vi "JIL-XML.vi"() -> ()   [LabVIEW 2010]
panel:
  in  "UseAuthentication":bool
  in  "MaxClients":i32=6
  out "clients":i32
  out "RegText":string
  in  "OpenFP":bool=TRUE
  out "error out 2":errorcluster={"status"=TRUE, "code"=56, "source"="TCP Wait On Listener in JIL-XML.vi"}
  in  "OpenParser":bool=TRUE
  out "error out":errorcluster
  out "Error":errorcluster={"status"=TRUE, "code"=56, "source"="TCP Wait On Listener in JIL-XML.vi"}
  in  "stop":bool=TRUE
  out "remote address":string
  in  "port":u16=2055
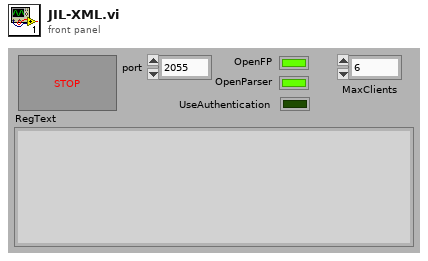
[diagram p1: front panel]
types:
  T1 = enum16{"Update", "registry", "Init", "clean", "Close"}
  T2 = enum32{"Invalid", "Standard", "Closed", "Hidden", "Minimized", "Maximized"}
  T3 = cluster{"remote address":string, "remote port":u16}
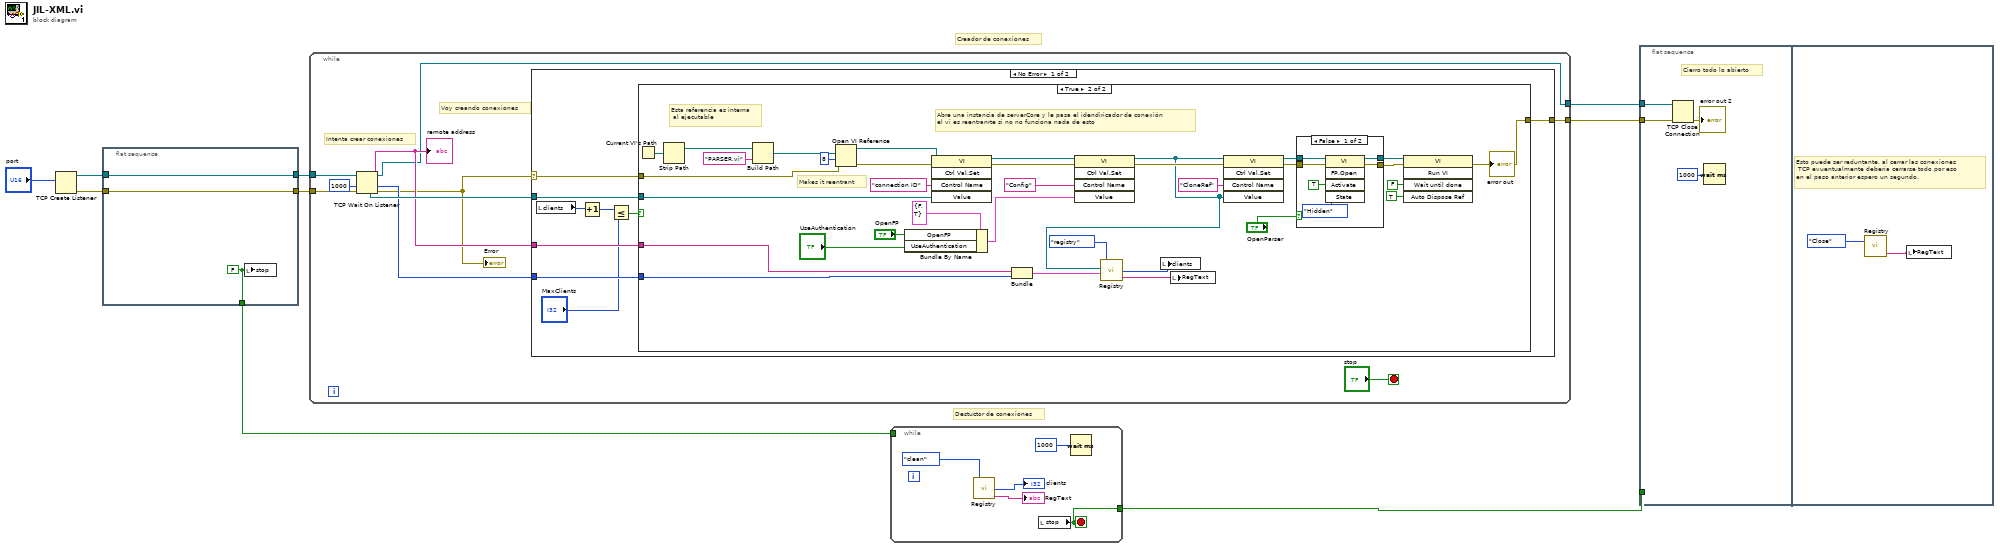
[diagram p0: block diagram]
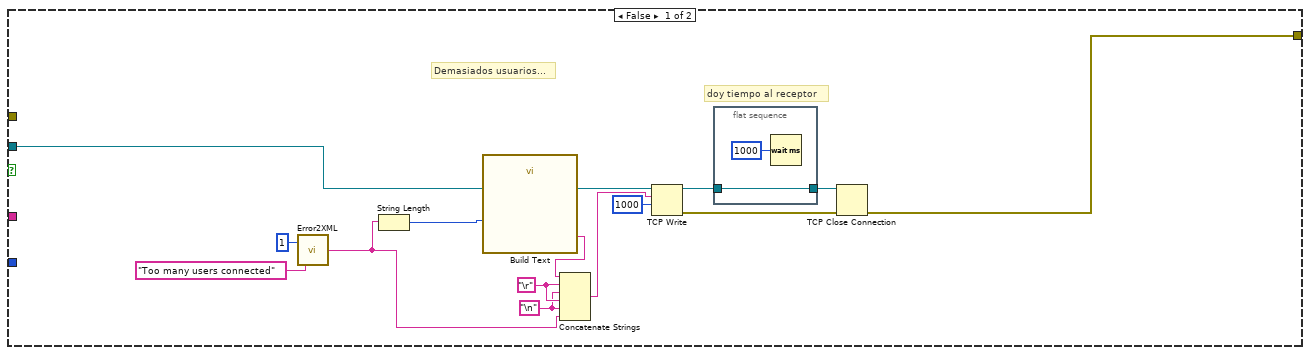
[diagram p2: hidden frame]
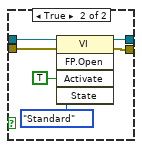
[diagram p3: hidden frame]
diagram:
  # "Destuctor de conexiones"
  # "Creador de conexiones"
  n1 = TCP Create Listener(10:"port") -> (0:w6:errorcluster, 3:w7:refnum<k5>)  [unwired: 4 in, 1 out]
  n2 = flat-sequence {
    tunnel: [w12] -> w8
    tunnel: w7 -> [w12]
    tunnel: w6 -> [w11]
    tunnel: [w11] -> w5
    tunnel: [w10] -> w3
    frame #0 {
      w10 = FALSE ("stop")
      n3 = local write "stop"(w10) -> ()
    }
  }
  n4 = while {
    tunnel: w8 -> [w15]
    tunnel: w5 -> [w22]
    tunnel: [w14] -> w1
    tunnel: [w18] -> w2
    stop <- "stop" stop-if-true
    # "Intenta crear conexiones"
    # "Voy creando conexiones"
    n5 = TCP Wait On Listener(8:w22, 9:1000 ("timeout ms (wait forever: -1)"), 11:w15) -> (0:w13:errorcluster, 1:w16:u16, 2:w17:string, 3:w14:refnum<k5>, 4:w21:refnum<k5>)  [unwired: 1 in]
    "remote address" <- w17
    "Error" <- w13
    n6 = case shown="No Error" w13 {
      selector: w13 -> [w27 w94]
      tunnel: w21 -> [w31 _]
      tunnel: [w30 w94] -> w18
      tunnel: w17 -> [w29 _]
      tunnel: w16 -> [w28 _]
      frame No Error {
        n7 = local read "clients"() -> (w24:i32)
        n8 = Increment(x=w24) -> (x+1=w25:i32)
        n9 = Less Or Equal?(x=w25, y="MaxClients") -> (x <= y?=w26:bool)
        n10 = case shown="True" w26 {
          tunnel: w31 -> [w42 w80]
          tunnel: [w40 w73] -> w30
          tunnel: w29 -> [_ w52]
          tunnel: w28 -> [_ w51]
          tunnel: w27 -> [_ w49]
          frame False {
            w34 = "\n"
            w35 = "\r"
            # "doy tiempo al receptor"
            # "Demasiados usuarios..."
            n11 = call "Error2XML.vi"("FailDescriptor"="Too many users connected", "FailID"=1) -> ("ErrorXML"=w32:string)
            n12 = String Length(string=w32) -> (length=w37:i32)
            n13 = call "Build Text"("longitud"=w37) -> ("Result"=w36:string)  [unwired: 13 in, 1 out]
            n14 = Concatenate Strings(w36, w35, w34, w35, w34, w32) -> (w33:string)
            n15 = TCP Write(connection ID=w42, data in=w33, 9:1000 ("timeout ms (25000)")) -> (connection ID out=w38:refnum<k5>, error out=w41:errorcluster)  [unwired: 1 in, 1 out]
            n16 = flat-sequence {
              tunnel: [w47] -> w39
              tunnel: w38 -> [w47]
              frame #0 {
                n17 = Wait (ms)(milliseconds to wait=u32 1000) -> ()  [unwired: 1 out]
              }
            }
            n18 = TCP Close Connection(connection ID=w39, error in (no error)=w41) -> (error out=w40:errorcluster)  [unwired: 1 in, 1 out]
          }
          frame True {
            # "Esta referencia es interna\n al ejecutable"
            # "Makes it reentrant"
            # "Abre una instancia de serverCore y le pasa el idendiricador de conexión\nel vi es reentranrte si no no funciona nada de esto"
            n19 = Current VI's Path() -> (path=w65:path)
            n20 = Strip Path(path=w65) -> (stripped path=w64:path)  [unwired: 1 out]
            n21 = Build Path(base path=w64, name or relative path="PARSER.vi") -> (appended path=w66:path)
            n22 = Open VI Reference(vi path=w66, options=8, error in (no error)=w49) -> (vi reference=w71:refnum<vi>, error out=w70:errorcluster)  [unwired: 3 in]
            n23 = Bundle By Name(cluster=cluster{"OpenFP":bool, "UseAuthentication":bool} {"OpenFP"=FALSE, "UseAuthentication"=TRUE} ("Config"), "OpenFP"="OpenFP", "UseAuthentication"="UseAuthentication") -> (w58:cluster{"OpenFP":bool, "UseAuthentication":bool})
            n24 = invoke class="VI" method="Ctrl Val.Set"(reference=w71, error in=w70, "Control Name"="connection ID", "Value"=w80) -> (reference out=w63:refnum<vi>, error out=w62:errorcluster)  [unwired: 1 in, 3 out]
            n25 = Bundle("remote address"=w52, "remote port"=w51) -> (w50:T3)  [unwired: 1 in]
            n26 = invoke class="VI" method="Ctrl Val.Set"(reference=w63, error in=w62, "Control Name"="Config", "Value"=w58) -> (reference out=w55:refnum<vi>, error out=w59:errorcluster)  [unwired: 1 in, 3 out]
            n27 = call "Registry.vi"("Client"=w50, "ParserReferecne"=w55, "Command"=T1."registry") -> ("RegText"=w53:string, "ConectionsNumber"=w48:i32)  [unwired: 1 in, 1 out]
            n28 = local write "clients"(w48) -> ()
            n29 = local write "RegText"(w53) -> ()
            n30 = invoke class="VI" method="Ctrl Val.Set"(reference=w55, error in=w59, "Control Name"="CloneRef", "Value"=w55) -> (reference out=w69:refnum<vi>, error out=w68:errorcluster)  [unwired: 1 in, 3 out]
            n31 = case shown="False" "OpenParser" {
              tunnel: w69 -> [w87 w93]
              tunnel: w68 -> [w85 w92]
              tunnel: [w86 w91] -> w78
              tunnel: [w84 w90] -> w77
              frame False {
                n32 = invoke class="VI" method="FP.Open"(reference=w87, error in=w85, "Activate"=TRUE ("Activate?"), "State"=T2."Hidden") -> (reference out=w86:refnum<vi>, error out=w84:errorcluster)  [unwired: 1 in, 3 out]
              }
              frame True {
                n33 = invoke class="VI" method="FP.Open"(reference=w93, error in=w92, "Activate"=TRUE ("Activate?"), "State"=T2."Standard") -> (reference out=w91:refnum<vi>, error out=w90:errorcluster)  [unwired: 1 in, 3 out]
              }
            }
            n34 = invoke class="VI" method="Run VI"(reference=w78, error in=w77, "Wait until done"=FALSE ("Wait Until Done"), "Auto Dispose Ref"=TRUE ("Auto Dispose Reference")) -> (error out=w73:errorcluster)  [unwired: 1 in, 4 out]
            "error out" <- w73
          }
        }
      }
      frame Error {
        # "Si no hay conexión no hago nada"
      }
    }
  }
  n35 = while {
    tunnel: [w98] -> w4
    tunnel: w3 -> [_]
    stop <- w98 stop-if-true
    n36 = call "Registry.vi"("Command"=T1."clean") -> ("RegText"=→"RegText":string, "ConectionsNumber"=→"clients":i32)  [unwired: 3 in, 1 out]
    n37 = local read "stop"() -> (w98:bool)
    n38 = Wait (ms)(milliseconds to wait=u32 1000) -> ()  [unwired: 1 out]
  }
  n39 = flat-sequence {
    tunnel: w1 -> [w102]
    tunnel: w2 -> [w101]
    tunnel: w4 -> [_]
    frame #0 {
      # "Cierro todo lo abierto"
      n40 = TCP Close Connection(connection ID=w102, error in (no error)=w101) -> (error out=→"error out 2":errorcluster)  [unwired: 1 in, 1 out]
      n41 = Wait (ms)(milliseconds to wait=u32 1000) -> ()  [unwired: 1 out]
    }
    frame #1 {
      # "Esto puede ser reduntante, al cerrar las conexiones\n TCP evuentualmente debería cerrarse todo por eso \nen el paso anterior espero un segundo."
      n42 = call "Registry.vi"("Command"=T1."Close") -> ("RegText"=w105:string)  [unwired: 3 in, 2 out]
      n43 = local write "RegText"(w105) -> ()
    }
  }
